vi "Untitled 1 (SubVI).vi"(10 "balls":T1[](array[typedef]), 11 "Robot in":T2) -> (3 "Robot out":T2)   [LabVIEW 2016]
uses:
  Core/AI Robot.ctl
  Core/AI Ball.ctl
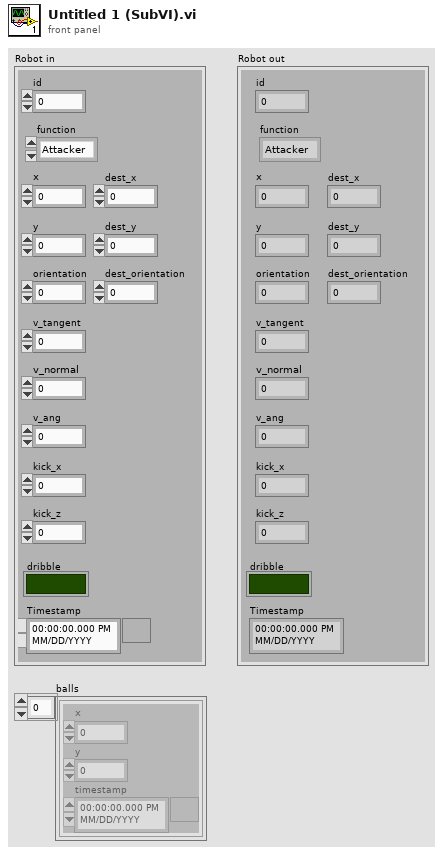
[diagram p1: front panel]
types:
  T1 = typedef "AI Ball.ctl" = cluster{"x":dbl, "y":dbl, "timestamp":timestamp}
  T2 = typedef "AI Robot.ctl" = cluster{"id":u32, "function":enum16{"Attacker", "Goalie", "Defender"}, "x":dbl, "y":dbl, "orientation":dbl, "v_tangent":dbl, "v_normal":dbl, "v_ang":dbl, "kick_x":dbl, "kick_z":dbl, "dribble":bool, "Timestamp":timestamp, "dest_x":dbl, "dest_y":dbl, "dest_orientation":dbl}
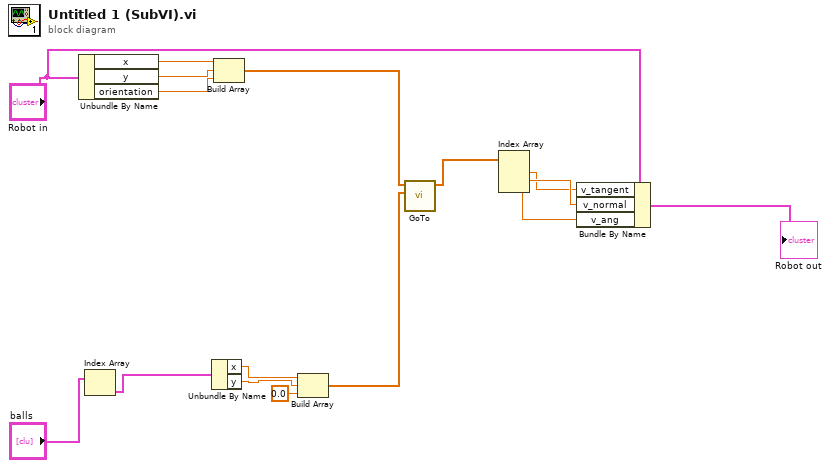
[diagram p0: block diagram]
diagram:
  n1 = Unbundle By Name("Robot in") -> ("x"=w1:dbl, "y"=w2:dbl, "orientation"=w3:dbl)
  n2 = Index Array(array="balls") -> (element=w6:T1)  [unwired: 1 in]
  n3 = Unbundle By Name(w6) -> ("x"=w8:dbl, "y"=w9:dbl)
  n4 = Build Array(w1, w2, w3) -> (w4:dbl[])
  n5 = Build Array(w8, w9, 0.0 ("element")) -> (w10:dbl[])
  n6 = call "GoTo.vi"("Target"=w10, "Position"=w4) -> ("Output\nVelocity"=w11:dbl[])  [unwired: 9 in]
  n7 = Index Array(array=w11) -> (element #1=w13:dbl, element #2=w14:dbl, element #3=w15:dbl)  [unwired: 3 in]
  n8 = Bundle By Name(cluster="Robot in", "v_tangent"=w13, "v_normal"=w14, "v_ang"=w15) -> (→"Robot out":T2)
